vi "OldFashionFXPWrite.vi"(8 "Error In":errorcluster) -> (0 "error out":errorcluster, 1 "Waveform Graph":dbl[](graph), 3 "Average":dbl)   [LabVIEW 2018]
uses:
  <vilib>/addons/FPGA Advanced Session Resources/LVFPGA Adv Session Resources/OpenByNameSubVI.vi
  <vilib>/rvi/interface/common/dynamic/niFpgaEscapeDelimiterAndNull.vi
  <vilib>/Utility/error.llb/Error Cluster From Error Code.vi
  <vilib>/rvi/errors/niLvFpgaAdjustHostInterfaceError.vi
  <vilib>/addons/FPGA Advanced Session Resources/LVFPGA Adv Session Resources/OpenByName.xnode
  <vilib>/rvi/interface/nirviReadWriteControl/nirviReadWriteControl.xnode
  NiFpgaLv.dll
  <vilib>/rvi/interface/Simulation/niFpgaSimulationCallBeginRW.vi
  <vilib>/addons/FPGA Advanced Session Resources/LVFPGA Adv Session Resources/LVFPGAAdvSessionResources.lvlib
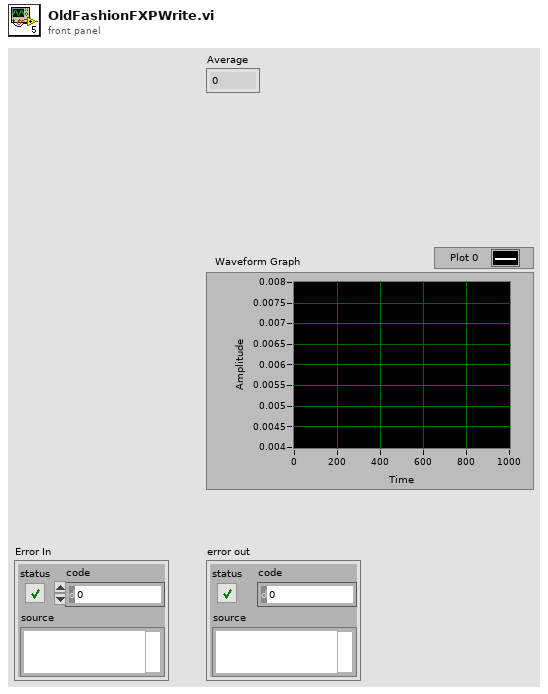
[diagram p1: front panel]
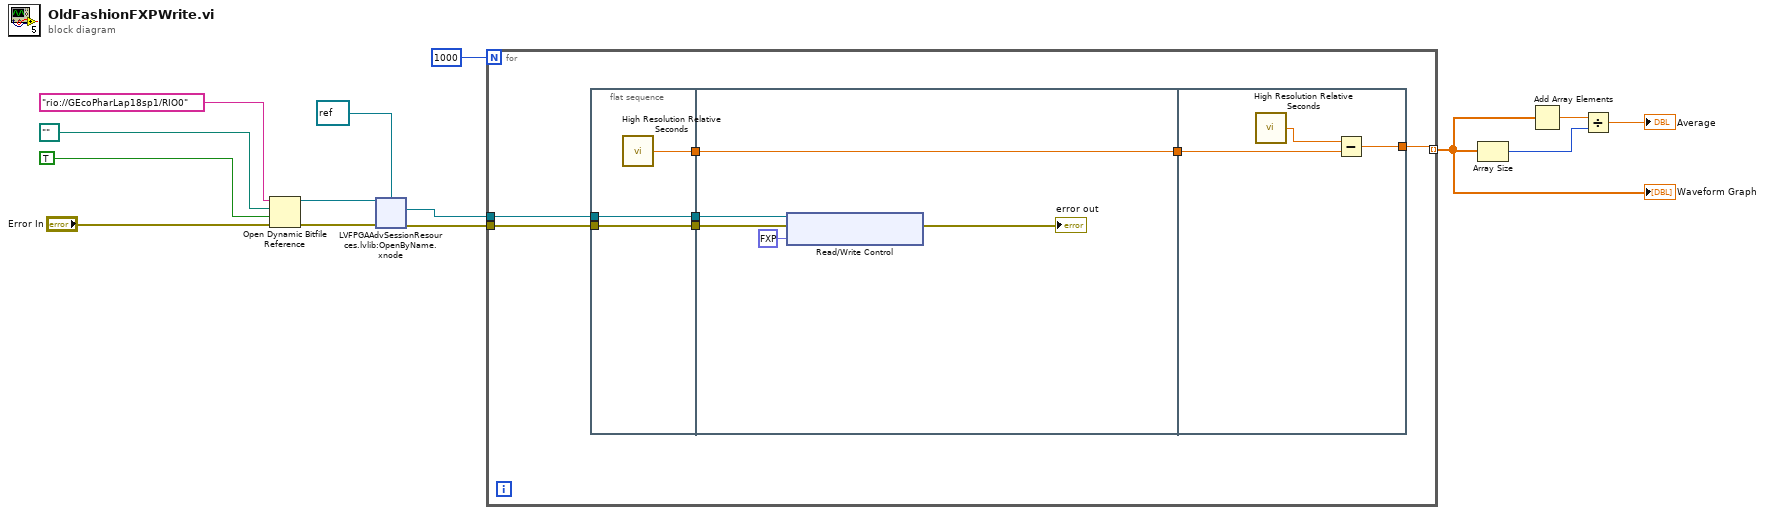
[diagram p0: block diagram]
diagram:
  n1 = Open Dynamic Bitfile Reference(0:"rio://GEcoPharLap18sp1/RIO0" ("Device address"), 1:path "" ("Bitfile path"), 2:TRUE ("Run When Loaded"), 3:"Error In") -> (5:w4:refnum<k20>, 8:w5:errorcluster)  [unwired: 1 in]
  n2 = xnode "LVFPGAAdvSessionResources.lvlib:OpenByName.xnode"("FPGA VI Reference in"=w4, "Single resource reference type in"=refnum<k20> refnum, "Error in"=w5) -> ("Single resource reference out"=w1:refnum<k20>, "Error out"=w2:errorcluster)  [unwired: 1 in, 1 out]
  n3 = for {
    N: 1000 -> [_]
    tunnel: [w19] -> w11 mode=indexing
    tunnel: w2 -> [w18]
    tunnel: w1 -> [w16]
    n4 = flat-sequence {
      tunnel: [w24] -> w21
      tunnel: w18 -> [w23]
      tunnel: [w23] -> w17
      tunnel: w16 -> [w22]
      tunnel: [w22] -> w15
      tunnel: w21 -> [w29]
      tunnel: [w29] -> w20
      tunnel: w17 -> [w28]
      tunnel: w15 -> [w27]
      tunnel: w20 -> [w31]
      tunnel: [w30] -> w19
      frame #0 {
        n5 = call <vilib>:"High Resolution Relative Seconds.vi"() -> ("relative seconds"=w24:dbl)
      }
      frame #1 {
        n6 = xnode "Read/Write Control"("FPGA VI Reference In"=w27, "error in"=w28, "1.5 Unsigned Indicator"=fxp<+,3,2> 1.0) -> ("error out"=→"error out":errorcluster)  [unwired: 1 out]
      }
      frame #2 {
        n7 = call <vilib>:"High Resolution Relative Seconds.vi"() -> ("relative seconds"=w32:dbl)
        n8 = Subtract(x=w32, y=w31) -> (x-y=w30:dbl)
      }
    }
  }
  "Waveform Graph" <- w11
  n9 = Array Size(array=w11) -> (size(s)=w13:i32)
  n10 = Add Array Elements(numeric array=w11) -> (sum=w14:dbl)
  n11 = Divide(x=w14, y=w13) -> (x/y=→"Average":dbl)
